vi "SetAllPaneSizes.vi"(8 "error in (no error)":errorcluster, 9 "Pane Sizes Array":i32[](array[numeric]), 10 "Pane position array":T1[](array[typedef])=[0, 1, 3, 4] items=["Top", "Left", "Center", "Right", "Bottom"], 11 "PentaPanesGUI in":refnum<class "PentaPanes.lvclass">) -> (0 "error out":errorcluster, 3 "PentaPanesGUI out":refnum<class "PentaPanes.lvclass">)   [LabVIEW 2022 SP3, in "PentaPanesLibrary.lvlib" / "PentaPanes.lvclass"]
uses:
  PentaPanes.lvclass
  PanePosition.ctl
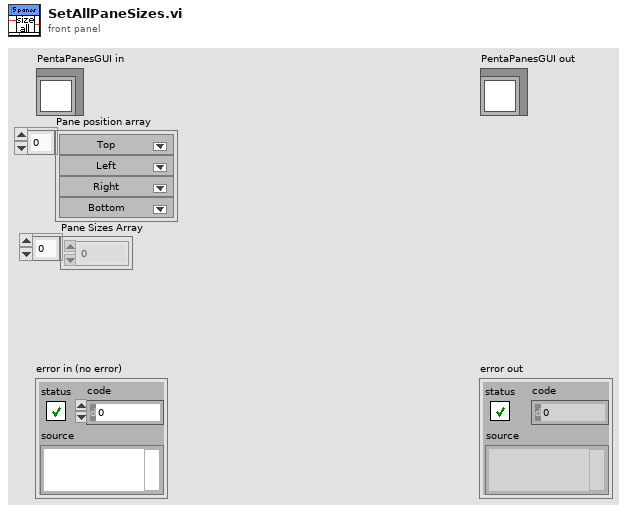
[diagram p1: front panel]
types:
  T1 = typedef "PentaPanesLibrary.lvlib/PentaPanes.lvclass/PanePosition.ctl" = u16
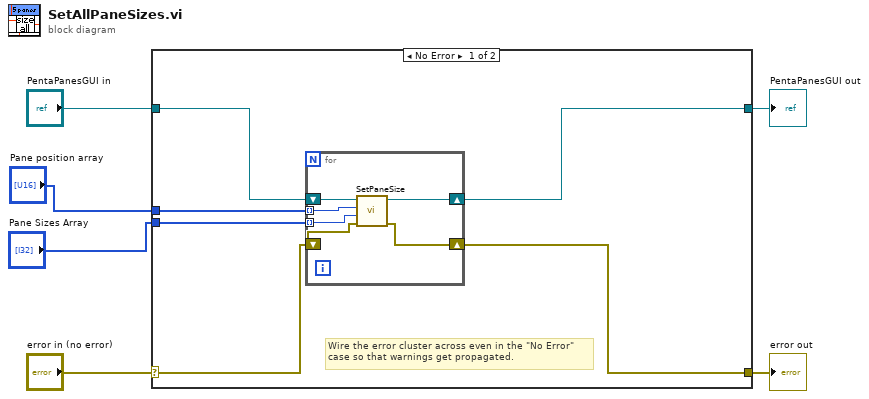
[diagram p0: block diagram]
diagram:
  n1 = case shown="No Error" "error in (no error)" {
    selector: "error in (no error)" -> [w8 w20]
    tunnel: [w7 w20] -> w5
    tunnel: [w12 w19] -> w3
    tunnel: "PentaPanesGUI in" -> [w11 w19]
    tunnel: "Pane position array" -> [w10 _]
    tunnel: "Pane Sizes Array" -> [w9 _]
    frame No Error {
      # "Wire the error cluster across even in the \"No Error\"\ncase so that warnings get propagated."
      n2 = for {
        shift-right: [w17] -> w12
        shift-left: w11 -> [w18]
        tunnel: w10 -> [w16] mode=indexing
        tunnel: w9 -> [w15] mode=indexing
        shift-right: [w13] -> w7
        shift-left: w8 -> [w14]
        n3 = call "SetPaneSize.vi"("error in (no error)"=w14, "Pane Size"=w15, "Pane Position"=w16, "PentaPanesGUI in"=w18) -> ("error out"=w13:errorcluster, "PentaPanesGUI out"=w17:refnum<class "PentaPanes.lvclass">)  [unwired: 6 in]
      }
    }
    frame Error {
    }
  }
  "error out" <- w5
  "PentaPanesGUI out" <- w3
